vi "globalTearDown.vi"(8 "error in (no error)":errorcluster, 11 "testcase-CSMSyncMessage in":refnum<class "testcase-CSMSyncMessage.lvclass">) -> (0 "error out":errorcluster, 3 "testcase-CSMSyncMessage out":refnum<class "testcase-CSMSyncMessage.lvclass">)   [LabVIEW 2017, in "testcase-CSMSyncMessage.lvclass"]
uses:
  testcase-CSMSyncMessage.lvclass
  src/user.lib/_NEVSTOP/Communicable State Machine(CSM)/_Support/Typedef/_CSM_List Module Scope.ctl
  src/user.lib/_NEVSTOP/Communicable State Machine(CSM)/Communicable State Machine.lvlib
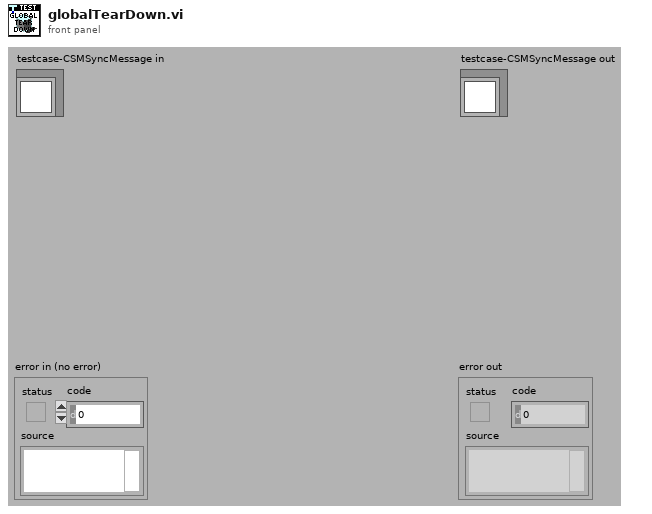
[diagram p1: front panel]
types:
  T1 = typedef "Communicable State Machine.lvlib/_CSM_List Module Scope.ctl" = enum16{"Normal", "System Only", "All"}
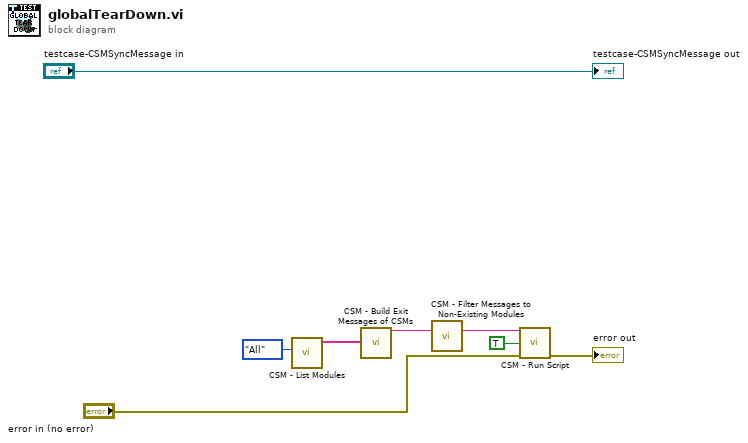
[diagram p0: block diagram]
diagram:
  n1 = call "CSM - List Modules.vi"("Scope (Normal)"=_CSM_List_Module_Scope."All") -> ("Module Names"=w2:string[])  [unwired: 9 in, 1 out]
  n2 = call "CSM - Build Exit Messages of CSMs.vi"("CSMs"=w2) -> ("States"=w8:string)  [unwired: 14 in]
  n3 = call "CSM - Filter Messages to Non-Existing Modules.vi"("State (S) In (\"\")"=w8) -> ("States Out"=w6:string)  [unwired: 14 in]
  n4 = call "CSM - Run Script.vi"("CSM Scripts"=w6, "Continue If Error? (F)"=TRUE, "error in (no error)"="error in (no error)") -> ("error out"=→"error out":errorcluster)  [unwired: 10 in, 2 out]
  "testcase-CSMSyncMessage out" <- "testcase-CSMSyncMessage in"
